vi "Format Bitpacked Array.vi"(10 "Length":i32, 11 "Value":u64) -> (3 "Array":i16[](array[numeric]))   [LabVIEW 2016, in "FPGA Addon Engine.lvlib"]
uses:
  FPGA Addon Engine.lvlib
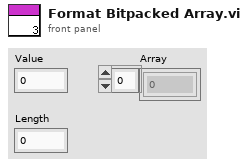
[diagram p1: front panel]
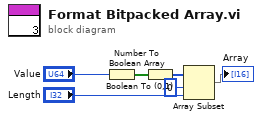
[diagram p0: block diagram]
diagram:
  n1 = Number To Boolean Array(number="Value") -> (Boolean array=w2:bool[])
  n2 = Boolean To (0,1)(Boolean=w2) -> (0, 1=w3:i16[])
  n3 = Array Subset(array=w3, index=0, length="Length") -> (→"Array":i16[])
